vi "SquareWave.vi"() -> ()   [LabVIEW 2012]
uses:
  <vilib>/rvi/eio/common/nirviEmuTemplateMethod_errors.vi
  <vilib>/eio/EIONode/EIONode.xnode
panel:
  in  "s":bool
  in  "offset":i16
  in  "duty cycle (periods)":fxp<+,32,0>=0.5
  in  "amplitude":i16=32767
  in  "frequency (periods/tick)":fxp<+,32,0>=0.0005000000819563866
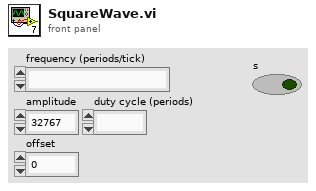
[diagram p1: front panel]
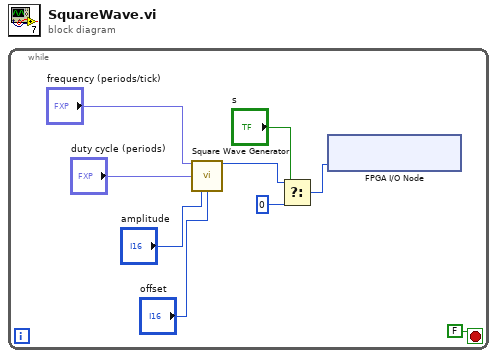
[diagram p0: block diagram]
diagram:
  n1 = while {
    stop <- FALSE ("stop") stop-if-true
    n2 = call "Square Wave Generator"("frequency (periods/tick)"="frequency (periods/tick)", "duty cycle (periods)"="duty cycle (periods)", "amplitude"="amplitude", "offset"="offset") -> ("square wave out"=w3:i16)  [unwired: 11 in]
    n3 = Select(t=w3, s="s", f=i16 0) -> (s? t:f=w1:i16)
    n4 = xnode "FPGA I/O Node"("Connector0/AO7"=w1) -> ()  [unwired: 1 in, 1 out]
  }
